vi "Communication Bus Template.Async.vi"(10 "Parameters":variant, 11 "Process":refnum<class "Process.lvclass">) -> ()   [LabVIEW 2020, in "Communication Bus Template Engine.lvlib"]
uses:
  Communication Bus Template Engine.lvlib
  <vilib>/NI/NIVS Inline Async API/_VS Inline Async API/Process/Process.lvclass
  Asynchronous Execution Unit Runtime Information.ctl
  <vilib>/NI/NIVS Inline Async API/_VS Inline Async API/Process/Process.lvclass/Process.ctl
  <vilib>/NI/NIVS Inline Async API/_Data Access Engine/Access Type Classes/Read/Read.lvclass/Read.ctl
  <vilib>/NI/NIVS Inline Async API/_Data Access Engine/Access Type Classes/Write/Write.lvclass/Write.ctl
  <vilib>/NI/NIVS Inline Async API/_Data Access Engine/Data Access Engine/Methods/Read.Data.vi
  <vilib>/NI/NIVS Inline Async API/_Data Access Engine/Data Access Engine/Methods/Write.Data.vi
  <vilib>/NI/NIVS Inline Async API/_VS Inline Async API/Process/Data Member Access/Read Data Access.vi
  <vilib>/NI/NIVS Inline Async API/_VS Inline Async API/Error Handling Process/SubVIs/Error.ConvertArray.vi
  <vilib>/NI/NIVS Inline Async API/_Data Access Engine/Access Type Classes/Read/Read.ProcessData.vi
  <vilib>/NI/NIVS Inline Async API/_Data Access Engine/Access Type Classes/Write/Write.ProcessData.vi
  <vilib>/NI/NIVS Inline Async API/_Data Access Engine/Access Type Classes/Write/Write.Buffer.vi
  <vilib>/NI/NIVS Inline Async API/_Data Access Engine/Access Type Classes/Write/Write.Commit.vi
  <vilib>/NI/NIVS Inline Async API/_Data Access Engine/Data Access Engine/Methods/Write.Lookup.vi
  <vilib>/NI/NIVS Inline Async API/_Data Access Engine/Data Access Engine/Methods/Read.Lookup.vi
  <vilib>/NI/NIVS Inline Async API/_Data Access Engine/Data Access Engine/Data Access Engine.lvclass
  Includes/Communication Bus Engine.lvlibp/Interfaces/Execution Unit/Execution Unit/Execution Unit.lvclass
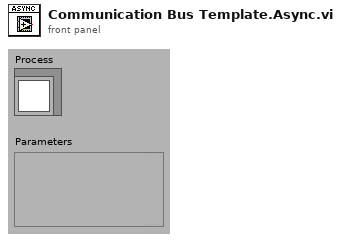
[diagram p1: front panel]
types:
  T1 = typedef "Communication Bus Template Engine.lvlib/Asynchronous Execution Unit Runtime Information.ctl" = cluster{"Execution Unit":refnum<class "Execution Unit.lvclass">, "Incoming Channel Group Name":string, "Outgoing Channel Group Name":string}
  T2 = typedef "Data Access Engine.lvlib/Data Access Engine.lvclass/Write.DVR.ctl" = refnum<data-value>
  T3 = typedef "Data Access Engine.lvlib/Data Access Engine.lvclass/Read.DVR.ctl" = refnum<data-value>
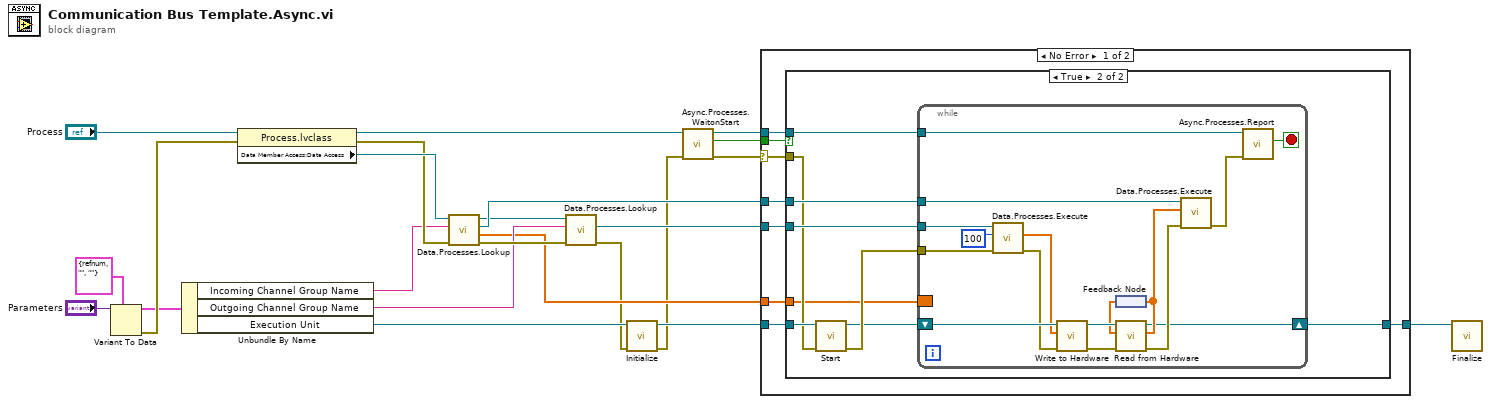
[diagram p0: block diagram]
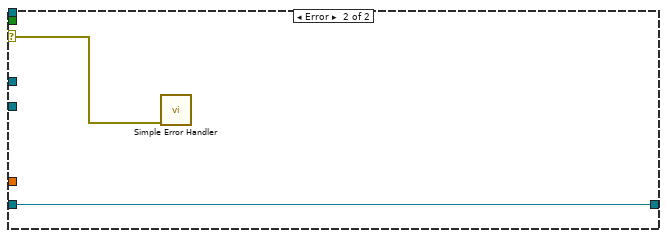
[diagram p3: hidden frame]
diagram:
  n1 = Variant To Data(type=T1 {"Execution Unit"=refnum, "Incoming Channel Group Name"="", "Outgoing Channel Group Name"=""} ("Asynchronous Execution Unit Runtime Information"), Variant="Parameters") -> (data=w9:T1, error out=w10:errorcluster)  [unwired: 1 in]
  n2 = Unbundle By Name(w9) -> ("Incoming Channel Group Name"=w8:string, "Outgoing Channel Group Name"=w7:string, "Execution Unit"=w5:refnum<class "Execution Unit.lvclass">)
  n3 = property class="Process.lvclass"(reference="Process", error in=w10) -> (reference out=w15:refnum<class "Process.lvclass">, error out=w13:errorcluster, "Data Member Access:Data Access"=w14:refnum<class "Data Access Engine.lvclass">)
  n4 = call-poly <vilib>:"Data.Processes.Lookup.vi"("error in (no error)"=w13, "Name"=w8, "Data Access API in"=w14) -> ("error out"=w19:errorcluster, "Initial Values"=w6:dbl[], "Ref"=w18:T2, "Data Access API out"=w17:refnum<class "Data Access Engine.lvclass">)  [unwired: 5 in]
  n5 = call-poly <vilib>:"Data.Processes.Lookup.vi"("error in (no error)"=w19, "Name"=w7, "Data Access API in"=w17) -> ("error out"=w3:errorcluster, "Ref"=w20:T3)  [unwired: 5 in, 2 out]
  n6 = call-dynamic "Initialize.vi"("error in (no error)"=w3, "Execution Unit in"=w5) -> ("error out"=w2:errorcluster, "Execution Unit out"=w4:refnum<class "Execution Unit.lvclass">)  [unwired: 8 in]
  n7 = call <vilib>:"Async.Processes.WaitonStart.vi"("error in (no error)"=w2, "Process"=w15) -> ("error out"=w21:errorcluster, "Execute"=w23:bool, "Process out"=w22:refnum<class "Process.lvclass">)  [unwired: 7 in]
  n8 = case shown="No Error" w21 {
    selector: w21 -> [w27 w59]
    tunnel: w23 -> [w31 _]
    tunnel: w22 -> [w30 _]
    tunnel: w18 -> [w29 _]
    tunnel: w20 -> [w28 _]
    tunnel: w6 -> [w26 _]
    tunnel: w4 -> [w25 w58]
    tunnel: [w24 w58] -> w1
    frame No Error {
      n9 = case shown="True" w31 {
        tunnel: w27 -> [_ w37]
        tunnel: w30 -> [_ w39]
        tunnel: w28 -> [_ w41]
        tunnel: w29 -> [_ w40]
        tunnel: w26 -> [_ w34]
        tunnel: w25 -> [w32 w38]
        tunnel: [w32 w33] -> w24
        frame False {
        }
        frame True {
          n10 = call-dynamic "Start.vi"("error in (no error)"=w37, "Execution Unit in"=w38) -> ("error out"=w36:errorcluster, "Execution Unit out"=w35:refnum<class "Execution Unit.lvclass">)  [unwired: 8 in]
          n11 = while {
            tunnel: w36 -> [w53]
            tunnel: w39 -> [w57]
            tunnel: w41 -> [w55]
            tunnel: w40 -> [w54]
            border: w34 -> [_]
            shift-right: [w42] -> w33
            shift-left: w35 -> [w51]
            stop <- w56 stop-if-true
            n12 = call-poly <vilib>:"Data.Processes.Execute.vi"("error in (no error)"=w53, "timeout ms"=100, "Ref"=w55) -> ("error out"=w48:errorcluster, "Values"=w49:dbl[])  [unwired: 6 in, 1 out]
            n13 = call-dynamic "Write to Hardware.vi"("error in (no error)"=w48, "Values in"=w49, "Execution Unit in"=w51) -> ("error out"=w47:errorcluster, "Execution Unit out"=w50:refnum<class "Execution Unit.lvclass">)  [unwired: 6 in, 1 out]
            n14 = feedback #1() -> (w44:dbl[])
            n15 = call-dynamic "Read from Hardware.vi"("error in (no error)"=w47, "Values in"=w44, "Execution Unit in"=w50) -> ("error out"=w46:errorcluster, "Values out"=w43:dbl[], "Execution Unit out"=w42:refnum<class "Execution Unit.lvclass">)  [unwired: 6 in]
            n16 = feedback-in #1(w43) -> ()
            n17 = call-poly <vilib>:"Data.Processes.Execute.vi"("error in (no error)"=w46, "Values"=w43, "Ref"=w54) -> ("error out"=w45:errorcluster)  [unwired: 8 in]
            n18 = call <vilib>:"Async.Processes.Report.vi"("Error"=w45, "Process in"=w57) -> ("Stop"=w56:bool)  [unwired: 8 in, 1 out]
          }
        }
      }
    }
    frame Error {
      n19 = call <vilib>:"Simple Error Handler.vi"("error in (no error)"=w59) -> ()  [unwired: 4 in, 5 out]
    }
  }
  n20 = call-dynamic "Finalize.vi"("Execution Unit in"=w1) -> ()  [unwired: 9 in, 2 out]
